vi "Daubechies4 Function.vi"(2 "iterations":u32=10, 3 "number of steps":i32=128) -> (0 "error":i32, 1 "Daubechies4 Function":dbl[](array[numeric]) format="%.2f")   [LabVIEW 2010, in "NI_Gmath.lvlib"]
doc: "The Daubechies4 function is calculated at evenly spaced sampled points."
uses:
  NI_Gmath.lvlib
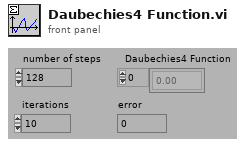
[diagram p1: front panel]
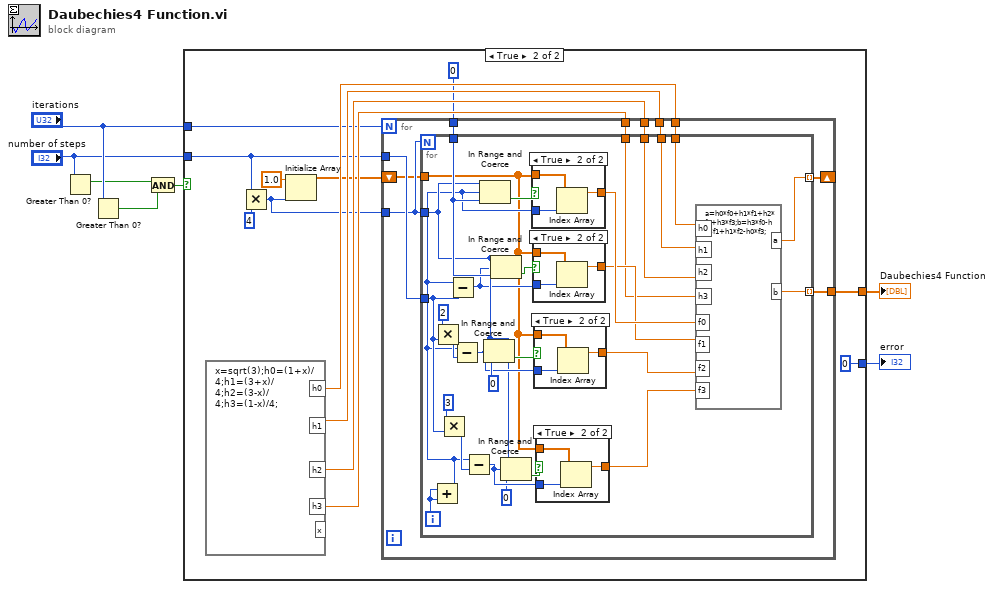
[diagram p0: block diagram]
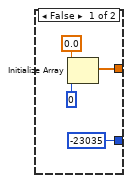
[diagram p2: hidden frame]
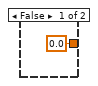
[diagram p3: hidden frame]
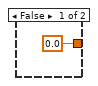
[diagram p4: hidden frame]
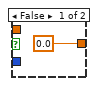
[diagram p5: hidden frame]
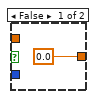
[diagram p6: hidden frame]
diagram:
  n1 = Greater Than 0?(x="number of steps") -> (x > 0?=w2:bool)
  n2 = Greater Than 0?(x="iterations") -> (x > 0?=w3:bool)
  n3 = And(x=w2, y=w3) -> (x .and. y?=w1:bool)
  n4 = case shown="True" w1 {
    tunnel: [w9 w24] -> w5
    tunnel: "number of steps" -> [_ w16]
    tunnel: "iterations" -> [_ w13]
    tunnel: [-23035 0] -> w4
    frame False {
      n5 = Initialize Array(0.0, 0) -> (w9:dbl[])
    }
    frame True {
      n6 = formula code="x=sqrt(3);h0=(1+x)/4;h1=(3+x)/4;h2=(3-x)/4;h3=(1-x)/4;"() -> ("h0"=w18:dbl, "h1"=w19:dbl, "h2"=w20:dbl, "h3"=w21:dbl)  [unwired: 1 out]
      n7 = Multiply(x=w16, y=4) -> (x*y=w15:i32)
      n8 = Initialize Array(1.0, w15) -> (w17:dbl[])
      n9 = for {
        N: w13 -> [_]
        shift-right: [w31] -> _
        shift-left: w17 -> [w25]
        tunnel: 0 -> [w34]
        tunnel: w15 -> [w32]
        tunnel: w16 -> [w33]
        tunnel: w18 -> [w30]
        tunnel: w19 -> [w29]
        tunnel: w20 -> [w28]
        tunnel: w21 -> [w27]
        tunnel: [w26] -> w24
        n10 = for {
          N: w32 -> [_]
          tunnel: w34 -> [w62]
          tunnel: w32 -> [w54]
          tunnel: w33 -> [w55]
          tunnel: [w46] -> w31 mode=indexing
          tunnel: w30 -> [w41]
          tunnel: w29 -> [w40]
          tunnel: w28 -> [w39]
          tunnel: w27 -> [w38]
          tunnel: [w37] -> w26 mode=indexing
          tunnel: w25 -> [w35]
          i -> [w43]
          n11 = Add(x=w43, y=w43) -> (x+y=w42:i32)
          n12 = Multiply(x=2, y=w55) -> (x*y=w45:i32)
          n13 = Multiply(x=3, y=w55) -> (x*y=w44:i32)
          n14 = Subtract(x=w42, y=w55) -> (x-y=w36:i32)
          n15 = Subtract(x=w42, y=w45) -> (x-y=w57:i32)
          n16 = Subtract(x=w42, y=w44) -> (x-y=w52:i32)
          n17 = In Range and Coerce(upper limit=w54, x=w42, lower limit=w62) -> (In Range?=w63:bool)  [unwired: 1 out]
          n18 = In Range and Coerce(upper limit=w54, x=w57, lower limit=0) -> (In Range?=w58:bool)  [unwired: 1 out]
          n19 = In Range and Coerce(upper limit=w54, x=w36, lower limit=w62) -> (In Range?=w61:bool)  [unwired: 1 out]
          n20 = In Range and Coerce(upper limit=w54, x=w52, lower limit=0) -> (In Range?=w53:bool)  [unwired: 1 out]
          n21 = case shown="True" w63 {
            tunnel: w35 -> [_ w79]
            tunnel: w42 -> [_ w78]
            tunnel: [0.0 w77] -> w50
            frame False {
            }
            frame True {
              n22 = Index Array(array=w79, index=w78) -> (element=w77:dbl)
            }
          }
          n23 = case shown="True" w61 {
            tunnel: w35 -> [_ w75]
            tunnel: w36 -> [_ w74]
            tunnel: [0.0 w73] -> w49
            frame False {
            }
            frame True {
              n24 = Index Array(array=w75, index=w74) -> (element=w73:dbl)
            }
          }
          n25 = case shown="True" w58 {
            tunnel: w35 -> [_ w71]
            tunnel: w57 -> [_ w70]
            tunnel: [0.0 w69] -> w48
            frame False {
            }
            frame True {
              n26 = Index Array(array=w71, index=w70) -> (element=w69:dbl)
            }
          }
          n27 = case shown="True" w53 {
            tunnel: w35 -> [_ w67]
            tunnel: w52 -> [_ w66]
            tunnel: [0.0 w65] -> w47
            frame False {
            }
            frame True {
              n28 = Index Array(array=w67, index=w66) -> (element=w65:dbl)
            }
          }
          n29 = formula code="a=h0*f0+h1*f1+h2*f2+h3*f3;b=h3*f0-h2*f1+h1*f2-h0*f3;"("h0"=w41, "h1"=w40, "h2"=w39, "h3"=w38, "f0"=w50, "f1"=w49, "f2"=w48, "f3"=w47) -> ("a"=w46:dbl, "b"=w37:dbl)
        }
      }
    }
  }
  "Daubechies4 Function" <- w5
  "error" <- w4
